vi "Get Size of Data from TD.vi"(8 "error in (no error)":errorcluster, 10 "Data String":u8[](array[numeric]), 11 "Type Descriptor":i16[](array[numeric])) -> (0 "error out":errorcluster, 2 "Size of Data":i32)   [LabVIEW 2017, in "Composition.lvlib"]
doc: "Returns the size of data of the <B>type descriptor</B> and <B>data string</B>."
uses:
  Composition.lvlib
  Get Data Type.vi/2a0888ac-0230-421b-a610-ddb651202d87.vi
  <vilib>/Utility/error.llb/Error Cluster From Error Code.vi
  <vilib>/ErrorRing/Error Ring.xnode
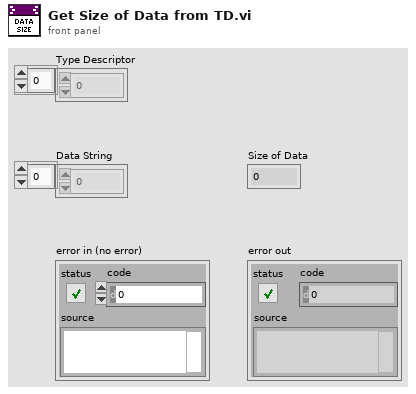
[diagram p1: front panel]
types:
  T1 = typedef "Composition.lvlib/Data Type.ctl" = enum16{"Void", "I8", "I16", "I32", "I64", "U8", "U16", "U32", "U64", "SGL", "DBL", "EXT", "CSG", "CDB", "CXT", "0x0F", "0x10", "0x11", "0x12", "0x13", "0x14", "Enum U8", "Enum U16", "Enum U32", "0x18", "SGL Physical", "DBL Physical", "EXT Physical", "CSG Physical", "CDB Physical", "CXT Physical", "0x1F", "Boolean U16", "Boolean U8", "0x22", "0x23", "0x24", "0x25", "0x26", "0x27", "0x28", "0x29", "0x2A", "0x2B", "0x2C", "0x2D", "0x2E", "0x2F", "String", "0x31", "Path", "Picture", "CString", "PString", "0x36", "Tag", "0x38", "0x39", "0x3A", "0x3B", "0x3C", "0x3D", "0x3E", "SubString", "Array", "Array Data Ptr", "0x42", "0x43", "0x44", "0x45", "0x46", "0x47", "0x48", "0x49", "0x4A", "0x4B", "0x4C", "0x4D", "0x4E", "SubArray", "Cluster", "0x51", "0x52", "Variant", "Waveform", "0x55", "0x56", "0x57", "0x58", "0x59", "0x5A", "0x5B", "0x5C", "0x5D", "CFX", "FXP", "Block", "Type Block", "Void Block", "Aligned Block", "Repeated Block", "Alignment Marker", "0x66", "0x67", "0x68", "0x69", "0x6A", "0x6B", "0x6C", "0x6D", "0x6E", "0x6F", "Refnum", "0x71", "0x72", "Set Collection", "Map Collection", "0x75", "0x76", "0x77", "0x78", "0x79", "0x7A", "0x7B", "0x7C", "0x7D", "0x7E", "0x7F", "Ptr", "0x81", "0x82", "Ptr to", "EXT Data", "0x85", "0x86", "0x87", "0x88", "0x89", "0x8A", "0x8B", "0x8C", "0x8D", "0x8E", "0x8F", "0x90", "0x91", "0x92", "0x93", "0x94", "0x95", "0x96", "0x97", "0x98", "0x99", "0x9A", "0x9B", "0x9C", "0x9D", "0x9E", "0x9F", "Array Interface", "Interface to Data", "0xA2", "0xA3", "0xA4", "0xA5", "0xA6", "0xA7", "0xA8", "0xA9", "0xAA", "0xAB", "0xAC", "0xAD", "0xAE", "0xAF", "0xB0", "0xB1", "0xB2", "0xB3", "0xB4", "0xB5", "0xB6", "0xB7", "0xB8", "0xB9", "0xBA", "0xBB", "0xBC", "0xBD", "0xBE", "0xBF", "0xC0", "0xC1", "0xC2", "0xC3", "0xC4", "0xC5", "0xC6", "0xC7", "0xC8", "0xC9", "0xCA", "0xCB", "0xCC", "0xCD", "0xCE", "0xCF", "0xD0", "0xD1", "0xD2", "0xD3", "0xD4", "0xD5", "0xD6", "0xD7", "0xD8", "0xD9", "0xDA", "0xDB", "0xDC", "0xDD", "0xDE", "0xDF", "0xE0", "0xE1", "0xE2", "0xE3", "0xE4", "0xE5", "0xE6", "0xE7", "0xE8", "0xE9", "0xEA", "0xEB", "0xEC", "0xED", "0xEE", "0xEF", "Function", "TypeDef", "PolyVI", "0xF3", "0xF4", "0xF5", "0xF6", "0xF7", "0xF8", "0xF9", "0xFA", "0xFB", "0xFC", "0xFD", "0xFE", "0xFF"}
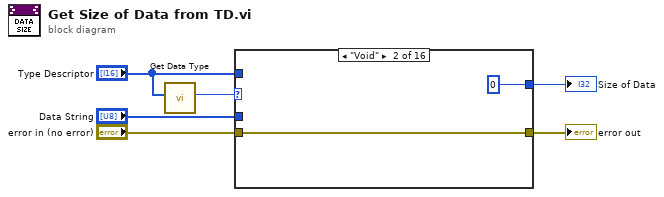
[diagram p0: block diagram]
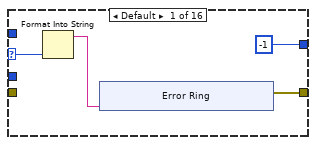
[diagram p2: hidden frame]
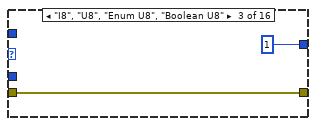
[diagram p3: hidden frame]
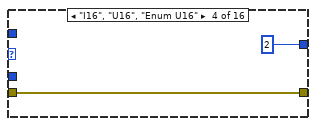
[diagram p4: hidden frame]
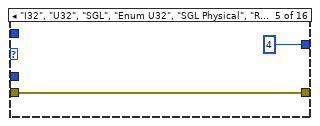
[diagram p5: hidden frame]
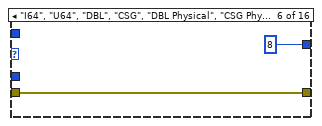
[diagram p6: hidden frame]
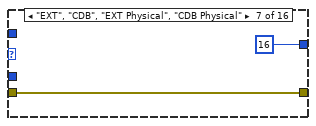
[diagram p7: hidden frame]
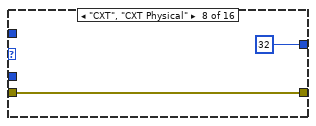
[diagram p8: hidden frame]
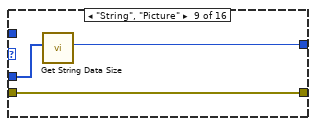
[diagram p9: hidden frame]
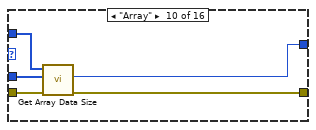
[diagram p10: hidden frame]
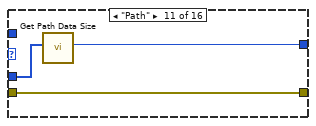
[diagram p11: hidden frame]
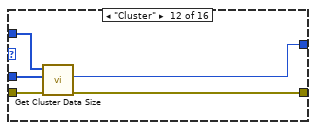
[diagram p12: hidden frame]
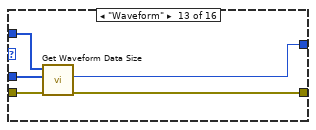
[diagram p13: hidden frame]
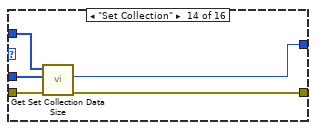
[diagram p14: hidden frame]
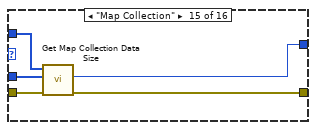
[diagram p15: hidden frame]
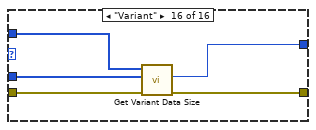
[diagram p16: hidden frame]
diagram:
  n1 = call "Get Data Type.vi"("Type Descriptor"="Type Descriptor") -> ("Data Type"=w3:T1)  [unwired: 10 in]
  n2 = case shown="\"Void\"" w3 {
    selector: w3 -> [w7 _ _ _ _ _ _ _ _ _ _ _ _ _ _ _]
    tunnel: "Data String" -> [_ _ _ _ _ _ _ _ w34 w38 w42 w46 w51 w56 w61 w64]
    tunnel: [-1 ("Data Size") 0 ("Size of Data") 1 ("Size of Data") 2 ("Size of Data") 4 ("Size of Data") 8 ("Size of Data") 16 ("Size of Data") 32 ("Size of Data") w33 w37 w41 w45 w50 w55 w60 w63] -> w5
    tunnel: "Type Descriptor" -> [_ _ _ _ _ _ _ _ _ w39 _ w47 w52 w57 w62 w65]
    tunnel: "error in (no error)" -> [_ w18 w20 w22 w24 w26 w28 w30 w32 w36 w40 w44 w49 w54 w59 w67]
    tunnel: [w8 w18 w20 w22 w24 w26 w28 w30 w32 w35 w40 w43 w48 w53 w58 w66] -> w1
    frame Default {
      n3 = Format Into String(w7) -> (resulting string=w9:string)  [unwired: 3 in, 1 out]
      n4 = xnode "Error Ring"("parameter 0"=w9) -> ("error out"=w8:errorcluster)
    }
    frame "Void" {
    }
    frame "I8", "U8", "Enum U8", "Boolean U8" {
    }
    frame "I16", "U16", "Enum U16" {
    }
    frame "I32", "U32", "SGL", "Enum U32", "SGL Physical", "Refnum" {
    }
    frame "I64", "U64", "DBL", "CSG", "DBL Physical", "CSG Physical" {
    }
    frame "EXT", "CDB", "EXT Physical", "CDB Physical" {
    }
    frame "CXT", "CXT Physical" {
    }
    frame "String", "Picture" {
      n5 = call "Get String Data Size.vi"("Data String"=w34) -> ("Data Size"=w33:i32)  [unwired: 10 in]
    }
    frame "Array" {
      n6 = call "Get Array Data Size.vi"("error in (no error)"=w36, "Data String"=w38, "Type Descriptor"=w39) -> ("error out"=w35:errorcluster, "Array Data Size"=w37:i32)  [unwired: 7 in]
    }
    frame "Path" {
      n7 = call "Get Path Data Size.vi"("Data String"=w42) -> ("Data Size"=w41:i32)  [unwired: 10 in]
    }
    frame "Cluster" {
      n8 = call "Get Cluster Data Size.vi"("error in (no error)"=w44, "Data String"=w46, "Type Descriptor"=w47) -> ("error out"=w43:errorcluster, "Data Size"=w45:i32)  [unwired: 7 in]
    }
    frame "Waveform" {
      n9 = call "Get Waveform Data Size.vi"("error in (no error)"=w49, "Data String"=w51, "Type Descriptor"=w52) -> ("error out"=w48:errorcluster, "Data Size"=w50:i32)  [unwired: 7 in]
    }
    frame "Set Collection" {
      n10 = call "Get Set Collection Data Size.vi"("error in (no error)"=w54, "Data String"=w56, "Type Descriptor"=w57) -> ("error out"=w53:errorcluster, "Data Size"=w55:i32)  [unwired: 7 in]
    }
    frame "Map Collection" {
      n11 = call "Get Map Collection Data Size.vi"("error in (no error)"=w59, "Data String"=w61, "Type Descriptor"=w62) -> ("error out"=w58:errorcluster, "Data Size"=w60:i32)  [unwired: 7 in]
    }
    frame "Variant" {
      n12 = call "Get Variant Data Size.vi"("error in (no error)"=w67, "Data String"=w64, "Type Descriptor"=w65) -> ("error out"=w66:errorcluster, "Data Size"=w63:i32)  [unwired: 7 in]
    }
  }
  "Size of Data" <- w5
  "error out" <- w1
